vi "Read_Finger_Position.vi"(8 "Error In":errorcluster, 11 "Leap Handle":T1) -> (0 "Error Out":errorcluster, 2 "Finger Positions":T2(array[cluster]), 3 "Leap Handle 2":T1)   [LabVIEW 2015]
uses:
  <vilib>/MakerHub/Leap/Private/Type Defs/Leap Handle.ctl
  C:/Program Files (x86)/National Instruments/LabVIEW 2015/vi.lib/MakerHub/Leap/Private/Libs/LeapCSharp.NET3.5.dll
  Program Files (x86)/National Instruments/LabVIEW 2015/vi.lib/MakerHub/Leap/Private/Libs/LeapCSharp.NET3.5.dll
  <vilib>/MakerHub/Leap/LMH-Leap.lvlib
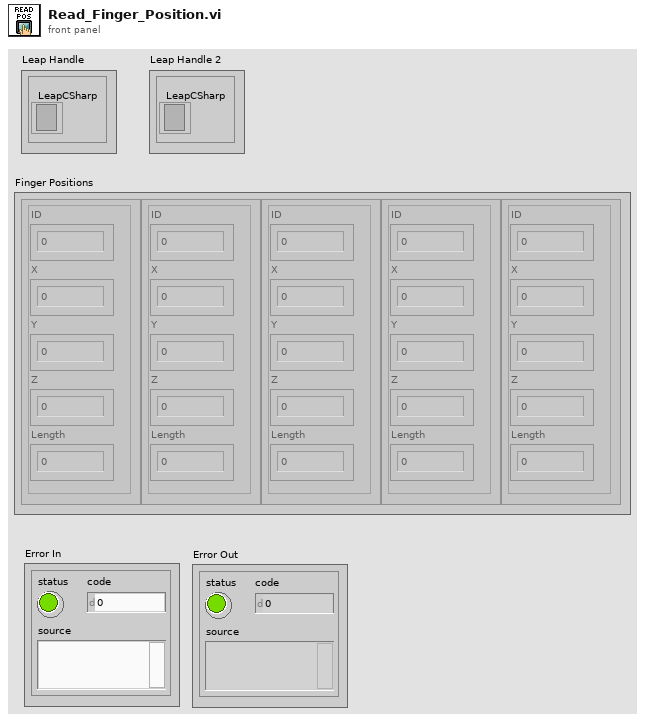
[diagram p1: front panel]
types:
  T1 = typedef "LMH-Leap.lvlib/Leap Handle.ctl" = cluster{"LeapCSharp":refnum<k24>}
  T2 = cluster{"ID":dbl, "X":dbl, "Y":dbl, "Z":dbl, "Length":dbl}[]
  T3 = typedef "LMH-Leap.lvlib/Frame.ctl" = cluster{"ID":i64, "Timestamp":i64, "Current FPS":dbl, "Key Tap Gestures":T4[], "Circle Gestures":T9[], "Screen Tap Gestures":T10[], "Swipe Gestures":T11[], "Hands":T12[]}
  T4 = typedef "LMH-Leap.lvlib/Gesture Key Tap.ctl" = cluster{"Common":T5, "Direction":T8, "Position":T8, "Progress":dbl}
  T5 = typedef "LMH-Leap.lvlib/Gesture Common.ctl" = cluster{"ID":dbl, "Duration (S)":dbl, "Gesture Type":T6, "Gesture State":T7}
  T6 = typedef "LMH-Leap.lvlib/Gesture Type.ctl" = enum16{"Invalid", "Swipe", "Circle", "Screen Tap", "Key Tap"}
  T7 = typedef "LMH-Leap.lvlib/Gesture State.ctl" = enum16{"Invalid", "Start", "Update", "Stop"}
  T8 = typedef "LMH-Leap.lvlib/Vector.ctl" = cluster{"Pitch":sgl, "Yaw":sgl, "Roll":sgl, "Magnitude":sgl, "XYZ":sgl[]}
  T9 = typedef "LMH-Leap.lvlib/Gesture Circle.ctl" = cluster{"Common":T5, "Center":T8, "Normal":T8, "Progress":dbl, "Radius":dbl}
  T10 = typedef "LMH-Leap.lvlib/Gesture Screen Tap.ctl" = cluster{"Common":T5, "Direction":T8, "Position":T8, "Progress":dbl}
  T11 = typedef "LMH-Leap.lvlib/Gesture Swipe.ctl" = cluster{"Common":T5, "Direction":T8, "Position":T8, "Start Position":T8, "Speed":dbl}
  T12 = typedef "LMH-Leap.lvlib/Hand.ctl" = cluster{"Palm Normal":T8, "Palm Position":T8, "Palm Velocity":T8, "Direction":T8, "Palm Position (Stabilized)":T8, "Sphere Center":T8, "Pointables":T13[], "ID":i32, "Time Visible":sgl, "Sphere Radius":sgl}
  T13 = typedef "LMH-Leap.lvlib/Pointable.ctl" = cluster{"Type":T14, "Touch Zone":T15, "ID":i32, "Length":dbl, "Width":dbl, "Time Visible":dbl, "Touch Distance":dbl, "Direction":T8, "Tip Position":T8, "Tip Velocity":T8, "Tip Position (Stabilized)":T8}
  T14 = typedef "LMH-Leap.lvlib/Pointable Type.ctl" = enum16{"Finger", "Tool"}
  T15 = typedef "LMH-Leap.lvlib/Pointable Zone.ctl" = enum16{"None", "Hovering", "Touching"}
  T16 = cluster{"ID":i32, "X":sgl, "Y":sgl, "Z":sgl, "Length":sgl}[]
  T17 = cluster{"ID":i32, "X":sgl, "Y":sgl, "Z":sgl, "Length":sgl}
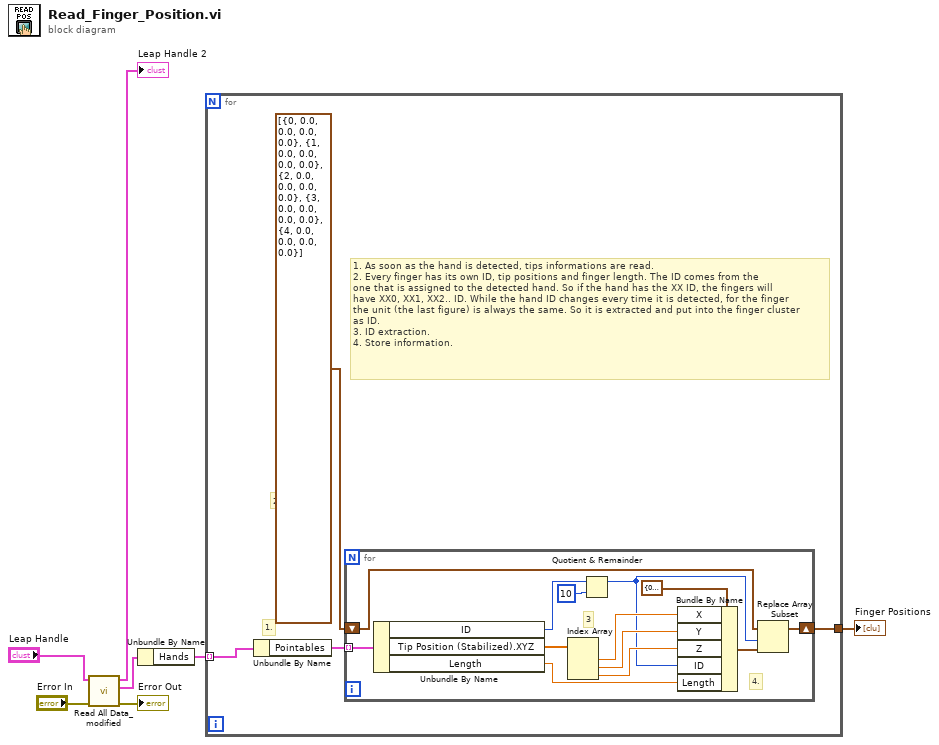
[diagram p0: block diagram]
diagram:
  n1 = call "Read All Data_modified.vi"("Error In"="Error In", "Leap Handle"="Leap Handle") -> ("Error Out"=→"Error Out":errorcluster, "Frame"=w2:T3, "Leap Handle"=→"Leap Handle 2":T1)  [unwired: 6 in, 1 out]
  n2 = Unbundle By Name(w2) -> ("Hands"=w7:T12[])
  n3 = for {
    tunnel: w7 -> [w11] mode=indexing
    tunnel: [w9] -> w6
    # "2."
    # "1."
    # "1. As soon as the hand is detected, tips informations are read.\n2. Every finger has its own ID, tip positions and finger length. The ID comes from the\none that is assigned to the detected hand. So if the hand has the XX ID, the fingers will\nhave XX0, XX1, XX2.. ID. While the hand ID changes every time it is detected, for the finger\nthe unit (the last figure) is always the same. So it is extracted and put into the finger cluster\nas ID.\n3. ID extraction.\n4. Store information."
    n4 = Unbundle By Name(w11) -> ("Pointables"=w10:T13[])
    n5 = for {
      tunnel: w10 -> [w19] mode=indexing
      shift-right: [w15] -> w9
      shift-left: T16 [{"ID"=0, "X"=0.0, "Y"=0.0, "Z"=0.0, "Length"=0.0}, {"ID"=1, "X"=0.0, "Y"=0.0, "Z"=0.0, "Length"=0.0}, {"ID"=2, "X"=0.0, "Y"=0.0, "Z"=0.0, "Length"=0.0}, {"ID"=3, "X"=0.0, "Y"=0.0, "Z"=0.0, "Length"=0.0}, {"ID"=4, "X"=0.0, "Y"=0.0, "Z"=0.0, "Length"=0.0}] -> [w16]
      # "4."
      # "3"
      n6 = Unbundle By Name(w19) -> ("ID"=w18:i32, "Tip Position (Stabilized).XYZ"=w23:sgl[], "Length"=w13:dbl)
      n7 = Index Array(array=w23) -> (element #1=w22:sgl, element #2=w21:sgl, element #3=w20:sgl)  [unwired: 3 in]
      n8 = Quotient & Remainder(x=w18, y=10) -> (x-y*floor(x/y)=w14:i32)  [unwired: 1 out]
      n9 = Bundle By Name(cluster=T17 {"ID"=0, "X"=0.0, "Y"=0.0, "Z"=0.0, "Length"=0.0}, "X"=w22, "Y"=w21, "Z"=w20, "ID"=w14, "Length"=w13) -> (w12:T17)
      n10 = Replace Array Subset(array=w16, new element=w12, index=w14) -> (w15:T16)
    }
  }
  "Finger Positions" <- w6
